vi "SelectMotorCommand.vi"(1 "Motor 1 Button Selector":T1(ring), 2 "Motor Amplitude":dbl) -> (0 "Motor Command":dbl)   [LabVIEW 2020]
uses:
  GlobalDriverStationCommands.vi
  GlobalDriverStationData.vi
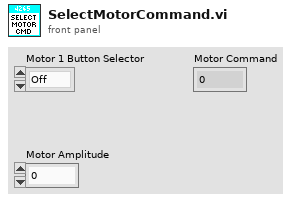
[diagram p1: front panel]
types:
  T1 = enum16{"Off", "Slider", "D_LT", "D_RT", "D_LB", "D_RB", "D_Y", "D_X", "D_A", "D_B", "M_LJoystick_X", "M_LJoystick_Y", "M_RJoystick_X", "M_RJoystick_Y", "M_LT", "M_RT", "M_LB", "M_RB", "M_Y", "M_X", "M_A", "M_B"}
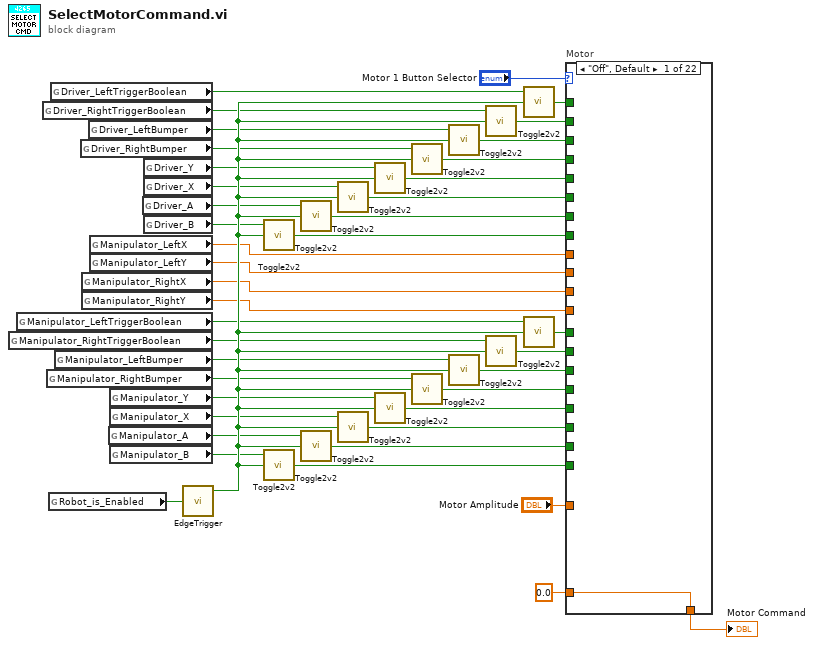
[diagram p0: block diagram]
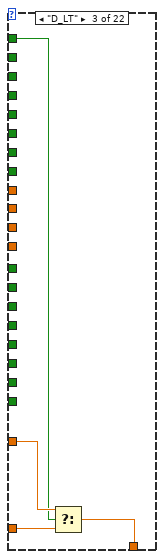
[diagram p3: hidden frame]
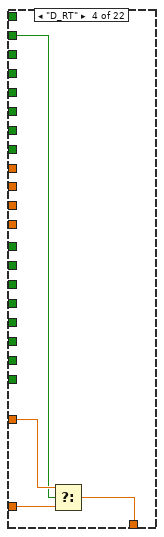
[diagram p4: hidden frame]
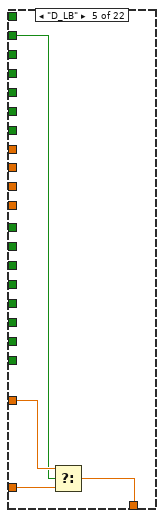
[diagram p5: hidden frame]
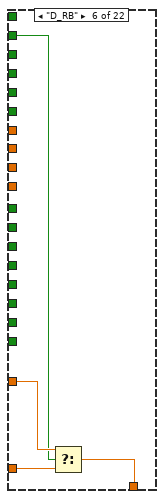
[diagram p6: hidden frame]
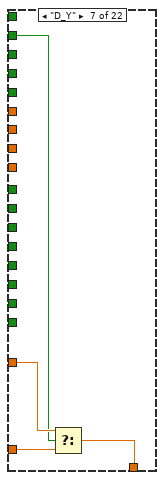
[diagram p7: hidden frame]
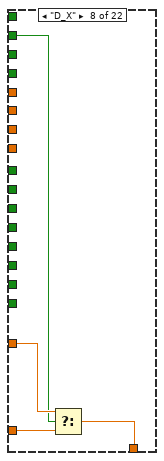
[diagram p8: hidden frame]
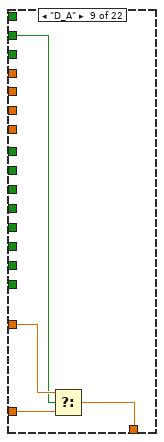
[diagram p9: hidden frame]
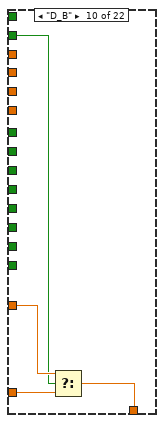
[diagram p10: hidden frame]
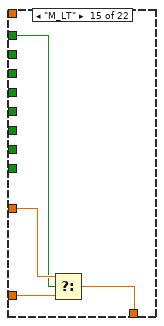
[diagram p15: hidden frame]
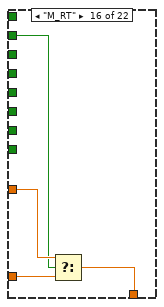
[diagram p16: hidden frame]
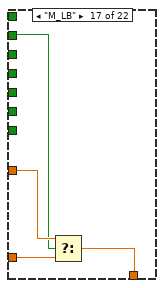
[diagram p17: hidden frame]
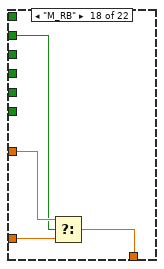
[diagram p18: hidden frame]
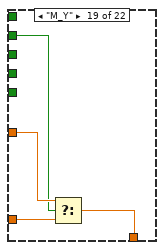
[diagram p19: hidden frame]
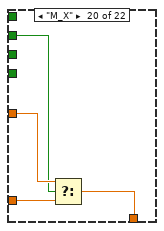
[diagram p20: hidden frame]
diagram:
  n1 = global read "GlobalDriverStationCommands.vi" "Manipulator_RightTriggerBoolean"() -> (w28:bool)
  n2 = global read "GlobalDriverStationCommands.vi" "Manipulator_LeftTriggerBoolean"() -> (w26:bool)
  n3 = global read "GlobalDriverStationCommands.vi" "Driver_RightTriggerBoolean"() -> (w12:bool)
  n4 = global read "GlobalDriverStationCommands.vi" "Manipulator_RightBumper"() -> (w32:bool)
  n5 = global read "GlobalDriverStationData.vi" "Robot_is_Enabled"() -> (w41:bool)
  n6 = global read "GlobalDriverStationCommands.vi" "Driver_LeftTriggerBoolean"() -> (w9:bool)
  n7 = global read "GlobalDriverStationCommands.vi" "Manipulator_LeftBumper"() -> (w30:bool)
  n8 = global read "GlobalDriverStationCommands.vi" "Driver_RightBumper"() -> (w15:bool)
  n9 = global read "GlobalDriverStationCommands.vi" "Manipulator_RightX"() -> (w3:dbl)
  n10 = global read "GlobalDriverStationCommands.vi" "Manipulator_RightY"() -> (w5:dbl)
  n11 = global read "GlobalDriverStationCommands.vi" "Driver_LeftBumper"() -> (w13:bool)
  n12 = global read "GlobalDriverStationCommands.vi" "Manipulator_LeftX"() -> (w2:dbl)
  n13 = global read "GlobalDriverStationCommands.vi" "Manipulator_LeftY"() -> (w4:dbl)
  n14 = global read "GlobalDriverStationCommands.vi" "Manipulator_A"() -> (w38:bool)
  n15 = global read "GlobalDriverStationCommands.vi" "Manipulator_Y"() -> (w33:bool)
  n16 = global read "GlobalDriverStationCommands.vi" "Manipulator_X"() -> (w36:bool)
  n17 = global read "GlobalDriverStationCommands.vi" "Manipulator_B"() -> (w40:bool)
  n18 = global read "GlobalDriverStationCommands.vi" "Driver_A"() -> (w22:bool)
  n19 = global read "GlobalDriverStationCommands.vi" "Driver_Y"() -> (w18:bool)
  n20 = global read "GlobalDriverStationCommands.vi" "Driver_X"() -> (w20:bool)
  n21 = global read "GlobalDriverStationCommands.vi" "Driver_B"() -> (w24:bool)
  n22 = call "EdgeTrigger.vi"("Input Signal"=w41) -> ("Rising Edge Trigger"=w42:bool)  [unwired: 2 out]
  n23 = call "Toggle2v2.vi"("Reset"=w42, "Trigger"=w24) -> ("New State"=w23:bool)  [unwired: 1 in]
  n24 = call "Toggle2v2.vi"("Reset"=w42, "Trigger"=w40) -> ("New State"=w39:bool)  [unwired: 1 in]
  n25 = call "Toggle2v2.vi"("Reset"=w42, "Trigger"=w22) -> ("New State"=w21:bool)  [unwired: 1 in]
  n26 = call "Toggle2v2.vi"("Reset"=w42, "Trigger"=w38) -> ("New State"=w37:bool)  [unwired: 1 in]
  n27 = call "Toggle2v2.vi"("Reset"=w42, "Trigger"=w20) -> ("New State"=w19:bool)  [unwired: 1 in]
  n28 = call "Toggle2v2.vi"("Reset"=w42, "Trigger"=w36) -> ("New State"=w35:bool)  [unwired: 1 in]
  n29 = call "Toggle2v2.vi"("Reset"=w42, "Trigger"=w18) -> ("New State"=w17:bool)  [unwired: 1 in]
  n30 = call "Toggle2v2.vi"("Reset"=w42, "Trigger"=w33) -> ("New State"=w34:bool)  [unwired: 1 in]
  n31 = call "Toggle2v2.vi"("Reset"=w42, "Trigger"=w15) -> ("New State"=w16:bool)  [unwired: 1 in]
  n32 = call "Toggle2v2.vi"("Reset"=w42, "Trigger"=w32) -> ("New State"=w31:bool)  [unwired: 1 in]
  n33 = call "Toggle2v2.vi"("Reset"=w42, "Trigger"=w13) -> ("New State"=w14:bool)  [unwired: 1 in]
  n34 = call "Toggle2v2.vi"("Reset"=w42, "Trigger"=w30) -> ("New State"=w29:bool)  [unwired: 1 in]
  n35 = call "Toggle2v2.vi"("Reset"=w42, "Trigger"=w12) -> ("New State"=w11:bool)  [unwired: 1 in]
  n36 = call "Toggle2v2.vi"("Reset"=w42, "Trigger"=w28) -> ("New State"=w27:bool)  [unwired: 1 in]
  n37 = call "Toggle2v2.vi"("Reset"=w42, "Trigger"=w9) -> ("New State"=w10:bool)  [unwired: 1 in]
  n38 = call "Toggle2v2.vi"("Reset"=w42, "Trigger"=w26) -> ("New State"=w25:bool)  [unwired: 1 in]
  n39 = case "Motor" shown="\"Off\", Default" "Motor 1 Button Selector" {
    tunnel: [w43 w44 w48 w52 w56 w60 w64 w68 w72 w76 w77 w78 w79 w80 w84 w88 w92 w96 w100 w104 w108 w112] -> w8
    tunnel: "Motor Amplitude" -> [_ w44 w47 w51 w55 w59 w63 w67 w71 w75 _ _ _ _ w83 w87 w91 w95 w99 w103 w107 w111]
    tunnel: w10 -> [_ _ w45 _ _ _ _ _ _ _ _ _ _ _ _ _ _ _ _ _ _ _]
    tunnel: w11 -> [_ _ _ w49 _ _ _ _ _ _ _ _ _ _ _ _ _ _ _ _ _ _]
    tunnel: w14 -> [_ _ _ _ w53 _ _ _ _ _ _ _ _ _ _ _ _ _ _ _ _ _]
    tunnel: w16 -> [_ _ _ _ _ w57 _ _ _ _ _ _ _ _ _ _ _ _ _ _ _ _]
    tunnel: w17 -> [_ _ _ _ _ _ w61 _ _ _ _ _ _ _ _ _ _ _ _ _ _ _]
    tunnel: w19 -> [_ _ _ _ _ _ _ w65 _ _ _ _ _ _ _ _ _ _ _ _ _ _]
    tunnel: w21 -> [_ _ _ _ _ _ _ _ w69 _ _ _ _ _ _ _ _ _ _ _ _ _]
    tunnel: w23 -> [_ _ _ _ _ _ _ _ _ w73 _ _ _ _ _ _ _ _ _ _ _ _]
    tunnel: w2 -> [_ _ _ _ _ _ _ _ _ _ w77 _ _ _ _ _ _ _ _ _ _ _]
    tunnel: w3 -> [_ _ _ _ _ _ _ _ _ _ _ _ w79 _ _ _ _ _ _ _ _ _]
    tunnel: w25 -> [_ _ _ _ _ _ _ _ _ _ _ _ _ _ w81 _ _ _ _ _ _ _]
    tunnel: w27 -> [_ _ _ _ _ _ _ _ _ _ _ _ _ _ _ w85 _ _ _ _ _ _]
    tunnel: w29 -> [_ _ _ _ _ _ _ _ _ _ _ _ _ _ _ _ w89 _ _ _ _ _]
    tunnel: w31 -> [_ _ _ _ _ _ _ _ _ _ _ _ _ _ _ _ _ w93 _ _ _ _]
    tunnel: w34 -> [_ _ _ _ _ _ _ _ _ _ _ _ _ _ _ _ _ _ w97 _ _ _]
    tunnel: w35 -> [_ _ _ _ _ _ _ _ _ _ _ _ _ _ _ _ _ _ _ w101 _ _]
    tunnel: w37 -> [_ _ _ _ _ _ _ _ _ _ _ _ _ _ _ _ _ _ _ _ w105 _]
    tunnel: w39 -> [_ _ _ _ _ _ _ _ _ _ _ _ _ _ _ _ _ _ _ _ _ w109]
    tunnel: 0.0 ("f") -> [w43 _ w46 w50 w54 w58 w62 w66 w70 w74 _ _ _ _ w82 w86 w90 w94 w98 w102 w106 w110]
    tunnel: w4 -> [_ _ _ _ _ _ _ _ _ _ _ w78 _ _ _ _ _ _ _ _ _ _]
    tunnel: w5 -> [_ _ _ _ _ _ _ _ _ _ _ _ _ w80 _ _ _ _ _ _ _ _]
    frame "Off", Default {
    }
    frame "Slider" {
    }
    frame "D_LT" {
      n40 = Select(t=w47, s=w45, f=w46) -> (s? t:f=w48:dbl)
    }
    frame "D_RT" {
      n41 = Select(t=w51, s=w49, f=w50) -> (s? t:f=w52:dbl)
    }
    frame "D_LB" {
      n42 = Select(t=w55, s=w53, f=w54) -> (s? t:f=w56:dbl)
    }
    frame "D_RB" {
      n43 = Select(t=w59, s=w57, f=w58) -> (s? t:f=w60:dbl)
    }
    frame "D_Y" {
      n44 = Select(t=w63, s=w61, f=w62) -> (s? t:f=w64:dbl)
    }
    frame "D_X" {
      n45 = Select(t=w67, s=w65, f=w66) -> (s? t:f=w68:dbl)
    }
    frame "D_A" {
      n46 = Select(t=w71, s=w69, f=w70) -> (s? t:f=w72:dbl)
    }
    frame "D_B" {
      n47 = Select(t=w75, s=w73, f=w74) -> (s? t:f=w76:dbl)
    }
    frame "M_LJoystick_X" {
    }
    frame "M_LJoystick_Y" {
    }
    frame "M_RJoystick_X" {
    }
    frame "M_RJoystick_Y" {
    }
    frame "M_LT" {
      n48 = Select(t=w83, s=w81, f=w82) -> (s? t:f=w84:dbl)
    }
    frame "M_RT" {
      n49 = Select(t=w87, s=w85, f=w86) -> (s? t:f=w88:dbl)
    }
    frame "M_LB" {
      n50 = Select(t=w91, s=w89, f=w90) -> (s? t:f=w92:dbl)
    }
    frame "M_RB" {
      n51 = Select(t=w95, s=w93, f=w94) -> (s? t:f=w96:dbl)
    }
    frame "M_Y" {
      n52 = Select(t=w99, s=w97, f=w98) -> (s? t:f=w100:dbl)
    }
    frame "M_X" {
      n53 = Select(t=w103, s=w101, f=w102) -> (s? t:f=w104:dbl)
    }
    frame "M_A" {
      n54 = Select(t=w107, s=w105, f=w106) -> (s? t:f=w108:dbl)
    }
    frame "M_B" {
      n55 = Select(t=w111, s=w109, f=w110) -> (s? t:f=w112:dbl)
    }
  }
  "Motor Command" <- w8
